vi "AlazarGetBoardRevision.vi"(0 "Handle":u64, 11 "error in (no error)":errorcluster) -> (4 "Handle":u64, 6 "Major Version":u8, 8 "Minor Version":u8, 10 "Return Code":u32, 15 "error out":errorcluster)   [LabVIEW 2009]
doc: "Get the PCB hadware revision level of a digitizer board."
uses:
  ATSApi.dll
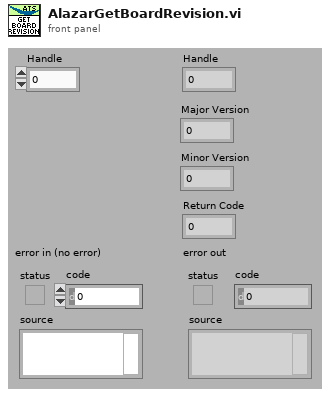
[diagram p1: front panel]
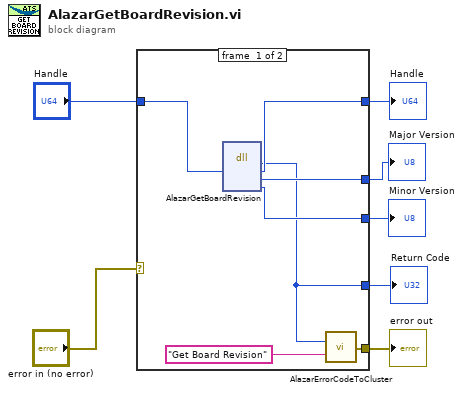
[diagram p0: block diagram]
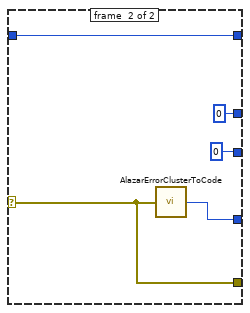
[diagram p2: hidden frame]
diagram:
  n1 = case shown="No Error" "error in (no error)" {
    selector: "error in (no error)" -> [_ w19]
    tunnel: [w10 w19] -> w6
    tunnel: [w9 w18] -> w5
    tunnel: "Handle" -> [w14 w17]
    tunnel: [w13 w17] -> w3
    tunnel: [w12 0] -> w2
    tunnel: [w11 0] -> w1
    frame #0 {
      n2 = dll-call lib="ATSApi.dll" fn="AlazarGetBoardRevision"("handle"=w14) -> ("return type"=w9:u32, "handle"=w13:u64, "majorVersion"=w12:u8, "minorVersion"=w11:u8)  [unwired: 5 in, 2 out]
      n3 = call "AlazarErrorCodeToCluster.vi"("Message"="Get Board Revision", "Error Code"=w9) -> ("error out"=w10:errorcluster)
    }
    frame #1 {
      n4 = call "AlazarErrorClusterToCode.vi"("error in (no error)"=w19) -> ("Error Code"=w18:u32)
    }
  }
  "Handle" <- w3
  "error out" <- w6
  "Return Code" <- w5
  "Major Version" <- w2
  "Minor Version" <- w1
